vi "Update.vi"(8 "error in (no error)":errorcluster, 10 "Message in":refnum<class "UpdateMessage.lvclass">, 11 "ConfocalStage in":refnum<class "ConfocalStage.lvclass">) -> (0 "error out":errorcluster, 3 "ConfocalStage out":refnum<class "ConfocalStage.lvclass">)   [LabVIEW 2012, in "ConfocalStage.lvclass"]
doc: "The update method processes the command 'update'. \n\nThe command 'update' is used for receiving new values to be set to the private data of the class. This could be seen as a public set method for setting new parameters to the private class data."
uses:
  ConfocalStage.lvclass
  <vilib>/Distrio/Murmex/UpdateMessage/UpdateMessage.lvclass
  ConfocalStage.lvclass/ConfocalStage.ctl
  <vilib>/Distrio/Murmex/Murmex/Murmex.lvclass
panel:
  # "This method is called when the UPDATE\ntrigger is sent. \n\nOverride this method when your component needs to\nrespond to this trigger. \n\nCall parent for proper implementation"
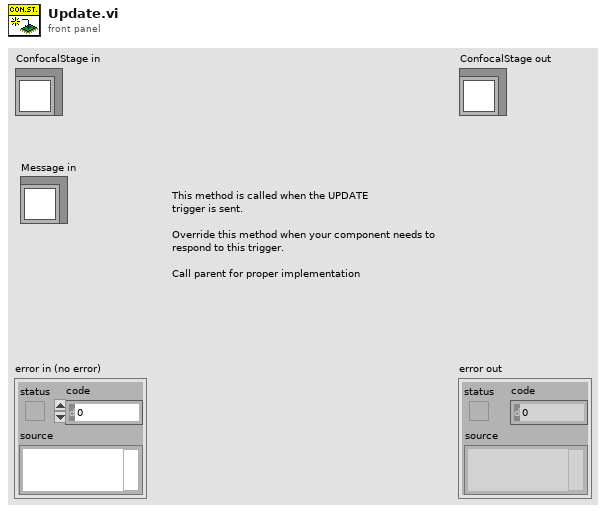
[diagram p1: front panel]
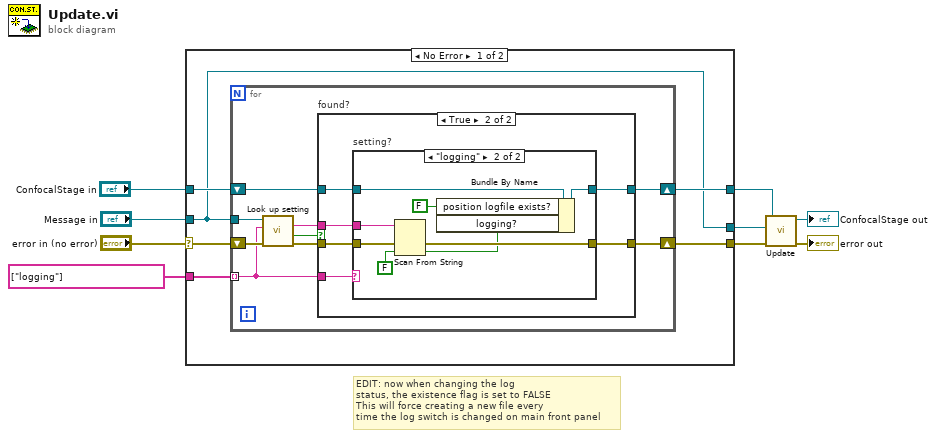
[diagram p0: block diagram]
diagram:
  # "EDIT: now when changing the log \nstatus, the existence flag is set to FALSE\nThis will force creating a new file every \ntime the log switch is changed on main front panel"
  n1 = case shown="No Error" "error in (no error)" {
    selector: "error in (no error)" -> [w14 w45]
    tunnel: [w11 w45] -> w6
    tunnel: [w10 w44] -> w5
    tunnel: "Message in" -> [w10 w44]
    tunnel: [w12 w43] -> w3
    tunnel: "ConfocalStage in" -> [w13 w43]
    tunnel: string[] ["logging"] ("key chains") -> [w15 _]
    frame No Error {
      n2 = for {
        tunnel: w15 -> [w19] mode=indexing
        tunnel: w10 -> [w23]
        shift-right: [w18] -> w11
        shift-left: w14 -> [w24]
        shift-right: [w16] -> w12
        shift-left: w13 -> [w17]
        n3 = call <vilib>:"Look up setting.vi"("error in (no error)"=w24, "tag name"=w19, "UpdateMessage in"=w23) -> ("error out"=w21:errorcluster, "found?"=w22:bool, "value"=w20:string)  [unwired: 5 in, 1 out]
        n4 = case "found?" shown="True" w22 {
          tunnel: w21 -> [w25 w31]
          tunnel: w20 -> [_ w30]
          tunnel: w19 -> [_ w32]
          tunnel: [w25 w29] -> w18
          tunnel: w17 -> [w26 w28]
          tunnel: [w26 w27] -> w16
          frame False {
          }
          frame True {
            n5 = case "setting?" shown="\"logging\"" w32 {
              tunnel: w31 -> [w33 w41]
              tunnel: w30 -> [_ w40]
              tunnel: [w33 w39] -> w29
              tunnel: w28 -> [w34 w38]
              tunnel: [w34 w36] -> w27
              frame "False", Default {
              }
              frame "logging" {
                n6 = Scan From String(input string=w40, error in=w41, default 1=FALSE ("settings.logging?")) -> (error out=w39:errorcluster, output 1=w37:bool)  [unwired: 2 in, 2 out]
                n7 = Bundle By Name(cluster=w38, "position logfile exists?"=FALSE ("runtime.position logfile exists?"), "logging?"=w37) -> (w36:refnum<class "ConfocalStage.lvclass">)
              }
            }
          }
        }
      }
    }
    frame Error {
    }
  }
  n8 = call-parent "Update.vi"("error in (no error)"=w6, "Message in"=w5, "Murmex in"=w3) -> ("error out"=→"error out":errorcluster, "Murmex out"=→"ConfocalStage out":refnum<class "ConfocalStage.lvclass">)  [unwired: 7 in]
